vi "Calculate Average Center.vi"(11 "Gantry Fiducials":dbl[](array[numeric])) -> (1 "Sensor ID Location":dbl[](array[numeric]), 2 "CH1 Location":dbl[](array[numeric]), 3 "XYZTheta":dbl[](array[numeric]))   [LabVIEW 2021, in "Component Tray.lvclass"]
uses:
  Component Tray.lvclass
  <vilib>/Analysis/baseanly.llb/Mean (DBL).vi
  <vilib>/Analysis/NI_AALBase.lvlib
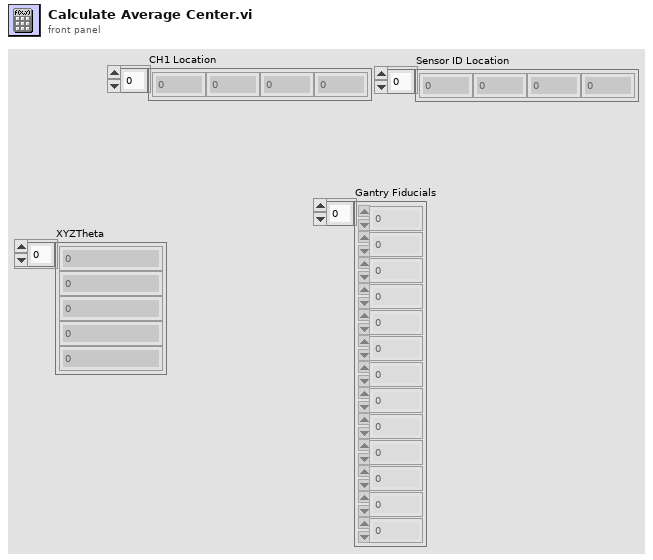
[diagram p1: front panel]
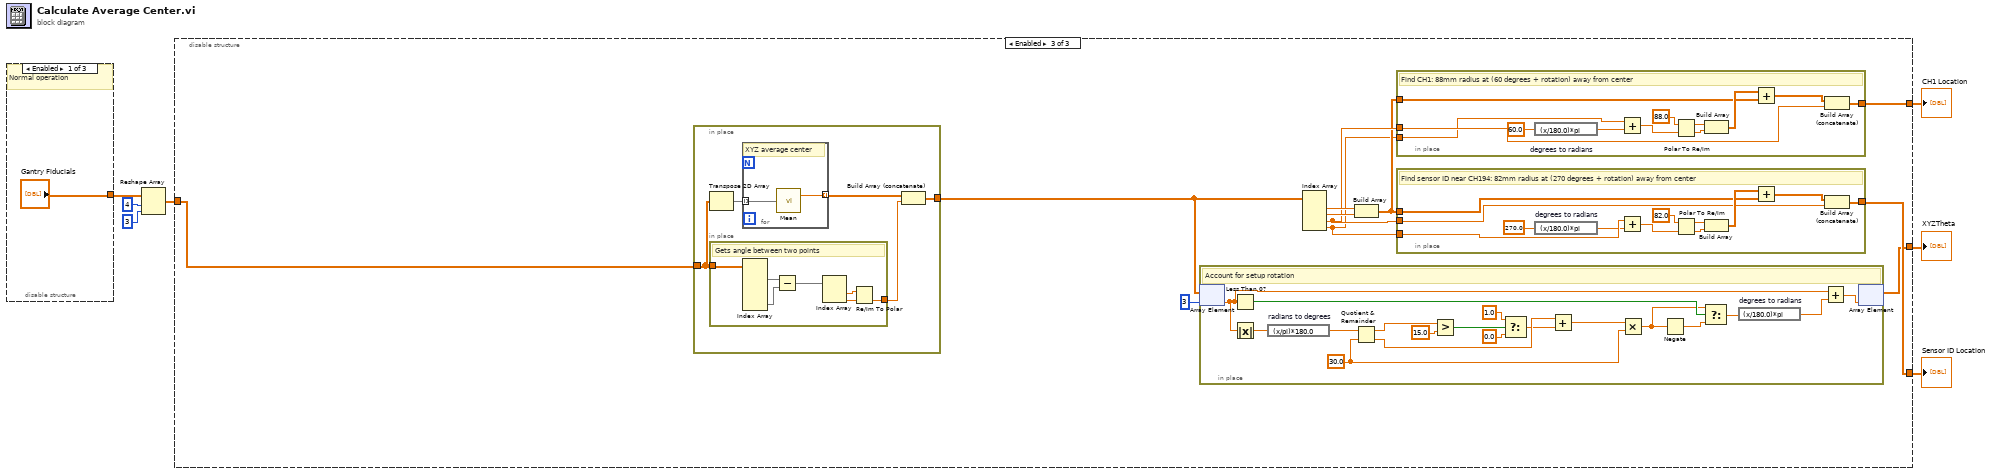
[diagram p0: block diagram]
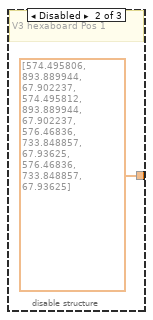
[diagram p2: hidden frame]
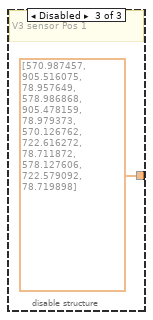
[diagram p3: hidden frame]
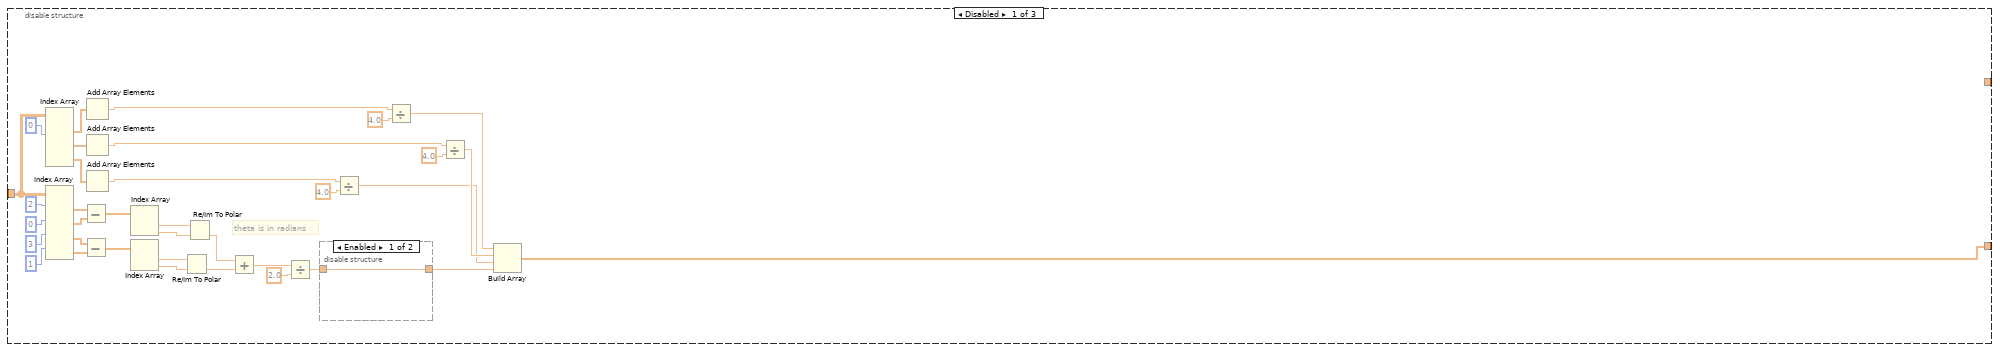
[diagram p4: hidden frame]
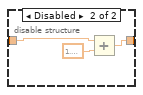
[diagram p5: hidden frame]
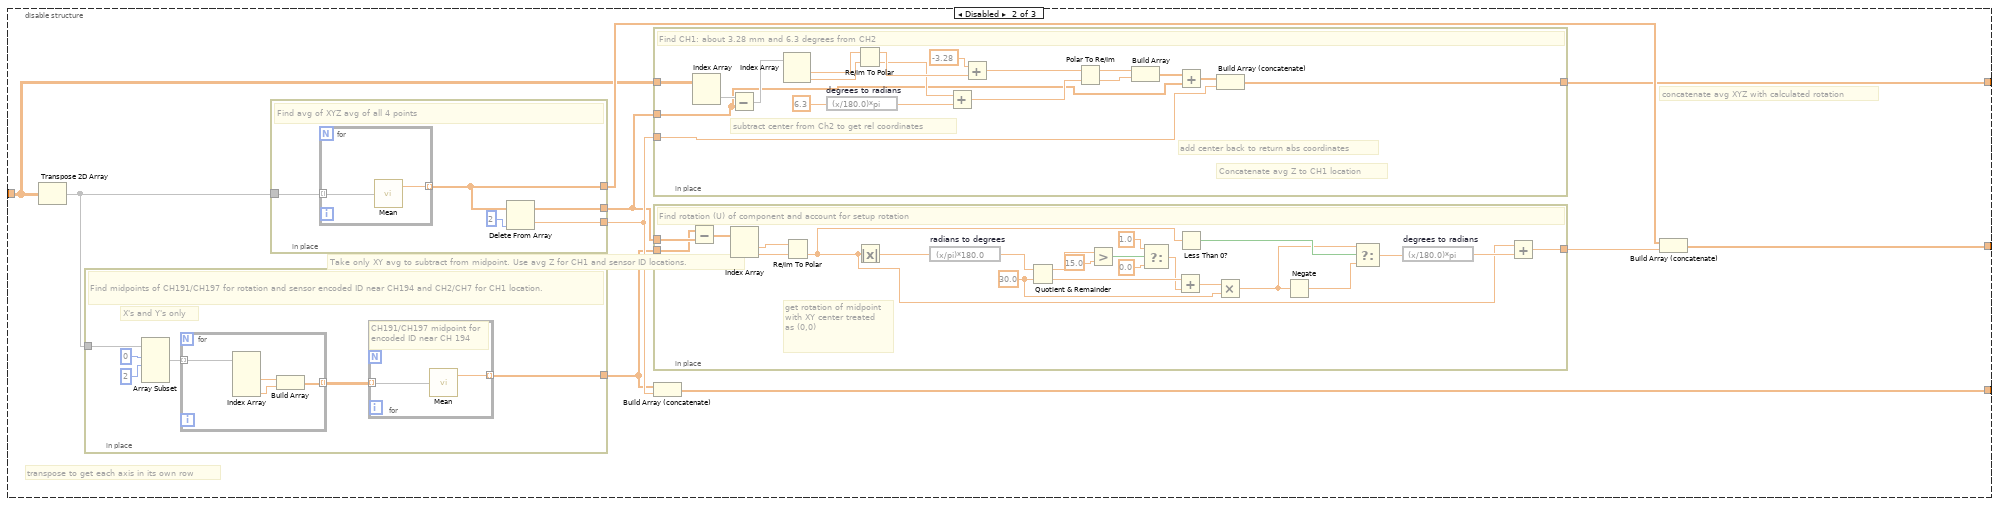
[diagram p6: hidden frame]
diagram:
  n1 = disable-structure shown="Enabled" {
    disable-tunnel: ["Gantry Fiducials" dbl[] [574.495806, 893.889944, 67.902237, 574.495812, 893.889944, 67.902237, 576.46836, 733.848857, 67.93625, 576.46836, 733.848857, 67.93625] dbl[] [570.987457, 905.516075, 78.957649, 578.986868, 905.478159, 78.979373, 570.126762, 722.616272, 78.711872, 578.127606, 722.579092, 78.719898]] -> w6
    frame Enabled {
      # "Normal operation"
    }
    frame Disabled {
      # "V3 hexaboard Pos 1"
    }
    frame Disabled {
      # "V3 sensor Pos 1"
    }
  }
  n2 = Reshape Array(w6, 4 ("dimension size"), 3 ("dimension size")) -> (w1:dbl[][])
  n3 = disable-structure shown="Enabled" {
    disable-tunnel: [w15 w59 w127] -> w7
    disable-tunnel: w1 -> [w14 w50 w129]
    disable-tunnel: [_ w55 w131] -> w5
    disable-tunnel: [_ w58 w130] -> w4
    frame Disabled {
      # "theta is in radians"
      n4 = Index Array(array=w14, index (col) #1=0 ("disabled index (col)")) -> (element #1=w44:dbl[], element #2=w43:dbl[], element #3=w13:dbl[])  [unwired: 5 in]
      n5 = Index Array(array=w14, index (row) #1=2 ("index (row)"), index (row) #2=0 ("index (row)"), index (row) #3=3 ("index (row)"), index (row) #4=1 ("index (row)")) -> (element #1=w28:dbl[], element #2=w27:dbl[], element #3=w26:dbl[], element #4=w25:dbl[])  [unwired: 4 in]
      n6 = Subtract(x=w28, y=w27) -> (x-y=w38:dbl[])
      n7 = Subtract(x=w26, y=w25) -> (x-y=w37:dbl[])
      n8 = Add Array Elements(numeric array=w44) -> (sum=w42:dbl)
      n9 = Add Array Elements(numeric array=w43) -> (sum=w41:dbl)
      n10 = Add Array Elements(numeric array=w13) -> (sum=w19:dbl)
      n11 = Index Array(array=w38) -> (element #1=w36:dbl, element #2=w35:dbl)  [unwired: 2 in]
      n12 = Index Array(array=w37) -> (element #1=w34:dbl, element #2=w33:dbl)  [unwired: 2 in]
      n13 = Re/Im To Polar(2:w33, 3:w34) -> (0:w31:dbl)  [unwired: 1 out]
      n14 = Re/Im To Polar(2:w35, 3:w36) -> (0:w32:dbl)  [unwired: 1 out]
      n15 = Add(x=w32, y=w31) -> (x+y=w30:dbl)
      n16 = Divide(x=w30, y=2.0) -> (x/y=w12:dbl)
      n17 = disable-structure shown="Enabled" {
        disable-tunnel: w12 -> [w46 w48]
        disable-tunnel: [w46 w47] -> w11
        frame Enabled {
        }
        frame Disabled {
          n18 = Add(x=w48, y=1.5707963267948966) -> (x+y=w47:dbl)
        }
      }
      n19 = Divide(x=w19, y=4.0) -> (x/y=w16:dbl)
      n20 = Divide(x=w42, y=4.0) -> (x/y=w18:dbl)
      n21 = Divide(x=w41, y=4.0) -> (x/y=w17:dbl)
      n22 = Build Array(w18, w17, w16, w11) -> (w15:dbl[])
    }
    frame Disabled {
      # "concatenate avg XYZ with calculated rotation"
      # "Take only XY avg to subtract from midpoint. Use avg Z for CH1 and sensor ID locations."
      # "transpose to get each axis in its own row"
      n23 = Transpose 2D Array(2D array=w50) -> (transposed array=w56:dbl[][])
      n24 = in-place {
        in-place-border: w56 -> [w107]
        in-place-border: [w102] -> w53
        # "X's and Y's only"
        # "Find midpoints of CH191/CH197 for rotation and sensor encoded ID near CH194 and CH2/CH7 for CH1 location."
        n25 = Array Subset(array=w107, index (row)=0 ("index"), length (row)=2 ("length")) -> (w104:dbl[][])  [unwired: 2 in]
        n26 = for {
          tunnel: w104 -> [w113] mode=indexing
          tunnel: [w110] -> w103 mode=indexing
          n27 = Index Array(array=w113) -> (element #2=w112:dbl, element #4=w111:dbl)  [unwired: 4 in, 2 out]
          n28 = Build Array(w112, w111) -> (w110:dbl[])
        }
        n29 = for {
          tunnel: [w108] -> w102 mode=indexing
          tunnel: w103 -> [w109] mode=indexing
          # "CH191/CH197 midpoint for encoded ID near CH 194"
          n30 = call-poly <vilib>:"Mean.vi"("X"=w109) -> ("mean"=w108:dbl)  [unwired: 1 out]
        }
      }
      n31 = in-place {
        in-place-border: w56 -> [w118]
        in-place-border: [w117] -> w57
        in-place-border: [w115] -> w54
        in-place-border: [w114] -> w52
        # "Find avg of XYZ avg of all 4 points"
        n32 = for {
          tunnel: [w120] -> w117 mode=indexing
          tunnel: w118 -> [w119] mode=indexing
          n33 = call-poly <vilib>:"Mean.vi"("X"=w119) -> ("mean"=w120:dbl)  [unwired: 1 out]
        }
        n34 = Delete From Array(array=w117, index=2) -> (deleted portion=w115:dbl, array with subset deleted=w114:dbl[])  [unwired: 1 in]
      }
      n35 = in-place {
        in-place-border: w52 -> [w62]
        in-place-border: w54 -> [w61]
        in-place-border: [w78] -> w55
        in-place-border: w50 -> [w76]
        # "add center back to return abs coordinates"
        # "subtract center from Ch2 to get rel coordinates"
        # "Concatenate avg Z to CH1 location"
        # "Find CH1: about 3.28 mm and 6.3 degrees from CH2"
        n36 = Index Array(array=w76) -> (element=w77:dbl[])  [unwired: 2 in]
        n37 = Subtract(x=w77, y=w62) -> (x-y=w75:dbl[])
        n38 = Index Array(array=w75) -> (element #1=w74:dbl, element #2=w73:dbl)  [unwired: 2 in]
        n39 = expression code="(x/180.0)*pi" "degrees to radians"(6.3) -> (w67:dbl)
        n40 = Re/Im To Polar(2:w73, 3:w74) -> (0:w68:dbl, 1:w71:dbl)
        n41 = Add(x=w68, y=w67) -> (x+y=w66:dbl)
        n42 = Add(x=-3.28 ("r"), y=w71) -> (x+y=w69:dbl)
        n43 = Polar To Re/Im(2:w66, 3:w69) -> (0:w64:dbl, 1:w65:dbl)
        n44 = Build Array(w65, w64) -> (w63:dbl[])
        n45 = Add(x=w63, y=w62) -> (x+y=w60:dbl[])
        n46 = Build Array (concatenate)(w60, w61) -> (w78:dbl[])
      }
      n47 = in-place {
        in-place-border: w52 -> [w98]
        in-place-border: w53 -> [w97]
        in-place-border: [w96] -> w51
        w81 = 30.0 ("y")
        # "get rotation of midpoint with XY center treated as (0,0)"
        # "Find rotation (U) of component and account for setup rotation"
        n48 = Subtract(x=w97, y=w98) -> (x-y=w99:dbl[])
        n49 = Index Array(array=w99) -> (element #1=w100:dbl, element #2=w101:dbl)  [unwired: 2 in]
        n50 = Re/Im To Polar(2:w101, 3:w100) -> (0:w80:dbl)  [unwired: 1 out]
        n51 = Absolute Value(x=w80) -> (abs(x)=w79:dbl)
        n52 = expression code="(x/pi)*180.0" "radians to degrees"(w79) -> (w93:dbl)
        n53 = Quotient & Remainder(x=w93, y=w81) -> (x-y*floor(x/y)=w86:dbl, floor(x/y)=w89:dbl)
        n54 = Greater?(x=w86, y=15.0) -> (0:w87:bool)
        n55 = Select(t=1.0, s=w87, f=0.0) -> (s? t:f=w88:dbl)
        n56 = Add(x=w89, y=w88) -> (x+y=w82:dbl)
        n57 = Less Than 0?(x=w80) -> (x < 0?=w94:bool)
        n58 = Multiply(x=w82, y=w81) -> (x*y=w91:dbl)
        n59 = Negate(x=w91) -> (-x=w92:dbl)
        n60 = Select(t=w91, s=w94, f=w92) -> (s? t:f=w90:dbl)
        n61 = expression code="(x/180.0)*pi" "degrees to radians"(w90) -> (w95:dbl)
        n62 = Add(x=w80, y=w95) -> (x+y=w96:dbl)
      }
      n63 = Build Array (concatenate)(w53, w54) -> (w58:dbl[])
      n64 = Build Array (concatenate)(w57, w51) -> (w59:dbl[])
    }
    frame Enabled {
      n65 = in-place {
        in-place-border: w129 -> [w146]
        in-place-border: [w145] -> w124
        n66 = Transpose 2D Array(2D array=w146) -> (transposed array=w148:dbl[][])
        n67 = in-place {
          in-place-border: [w153] -> w144
          in-place-border: w146 -> [w152]
          # "Gets angle between two points"
          n68 = Index Array(array=w152) -> (element #1=w151:dbl[], element #3=w149:dbl[])  [unwired: 6 in, 1 out]
          n69 = Subtract(x=w151, y=w149) -> (x-y=w150:dbl[])
          n70 = Index Array(array=w150) -> (element #1=w155:dbl, element #2=w154:dbl)  [unwired: 2 in]
          n71 = Re/Im To Polar(2:w154, 3:w155) -> (0:w153:dbl)  [unwired: 1 out]
        }
        n72 = for {
          tunnel: w148 -> [w157] mode=indexing
          tunnel: [w156] -> w147 mode=indexing
          # "XYZ average center"
          n73 = call-poly <vilib>:"Mean.vi"("X"=w157) -> ("mean"=w156:dbl)  [unwired: 1 out]
        }
        n74 = Build Array (concatenate)(w147, w144) -> (w145:dbl[])
      }
      n75 = in-place {
        w173 = 30.0 ("y")
        # "Account for setup rotation"
        n76 = in-place-array #1(w124, 3) -> (w170:dbl)
        n77 = Less Than 0?(x=w170) -> (x < 0?=w186:bool)
        n78 = Absolute Value(x=w170) -> (abs(x)=w172:dbl)
        n79 = expression code="(x/pi)*180.0" "radians to degrees"(w172) -> (w185:dbl)
        n80 = Quotient & Remainder(x=w185, y=w173) -> (x-y*floor(x/y)=w178:dbl, floor(x/y)=w181:dbl)
        n81 = Greater?(x=w178, y=15.0) -> (0:w179:bool)
        n82 = Select(t=1.0, s=w179, f=0.0) -> (s? t:f=w180:dbl)
        n83 = Add(x=w181, y=w180) -> (x+y=w174:dbl)
        n84 = Multiply(x=w174, y=w173) -> (x*y=w183:dbl)
        n85 = Negate(x=w183) -> (-x=w184:dbl)
        n86 = Select(t=w183, s=w186, f=w184) -> (s? t:f=w182:dbl)
        n87 = expression code="(x/180.0)*pi" "degrees to radians"(w182) -> (w187:dbl)
        n88 = Add(x=w170, y=w187) -> (x+y=w171:dbl)
        n89 = in-place-array #1(w171) -> (w127:dbl[])  [unwired: 1 out]
      }
      n90 = Index Array(array=w124) -> (element #1=w126:dbl, element #2=w125:dbl, element #3=w123:dbl, element #4=w121:dbl)  [unwired: 4 in]
      n91 = Build Array(w126, w125) -> (w122:dbl[])
      n92 = in-place {
        in-place-border: [w136] -> w131
        in-place-border: w123 -> [w134]
        in-place-border: w121 -> [w133]
        in-place-border: w122 -> [w132]
        # "Find CH1: 88mm radius at (60 degrees + rotation) away from center"
        n93 = expression code="(x/180.0)*pi" "degrees to radians"(60.0) -> (w142:dbl)
        n94 = Add(x=w133, y=w142) -> (x+y=w141:dbl)
        n95 = Polar To Re/Im(2:w141, 3:88.0 ("r")) -> (0:w139:dbl, 1:w140:dbl)
        n96 = Build Array(w140, w139) -> (w138:dbl[])
        n97 = Add(x=w138, y=w132) -> (x+y=w137:dbl[])
        n98 = Build Array (concatenate)(w137, w134) -> (w136:dbl[])
      }
      n99 = in-place {
        in-place-border: w122 -> [w165]
        in-place-border: [w162] -> w130
        in-place-border: w121 -> [w163]
        in-place-border: w123 -> [w161]
        # "Find sensor ID near CH194: 82mm radius at (270 degrees + rotation) away from center"
        n100 = expression code="(x/180.0)*pi" "degrees to radians"(270.0) -> (w160:dbl)
        n101 = Add(x=w163, y=w160) -> (x+y=w169:dbl)
        n102 = Polar To Re/Im(2:w169, 3:82.0 ("r")) -> (0:w167:dbl, 1:w168:dbl)
        n103 = Build Array(w168, w167) -> (w166:dbl[])
        n104 = Add(x=w166, y=w165) -> (x+y=w164:dbl[])
        n105 = Build Array (concatenate)(w164, w161) -> (w162:dbl[])
      }
    }
  }
  "XYZTheta" <- w7
  "CH1 Location" <- w5
  "Sensor ID Location" <- w4
